vi "String_conversions.vi"() -> ()   [LabVIEW 2019]
panel:
  in  "string 2":string
  out "all lower case string":string
  in  "string":string
  out "all upper case string":string
  in  "width (-)":i16
  in  "number":i32
  out "decimal integer string":string
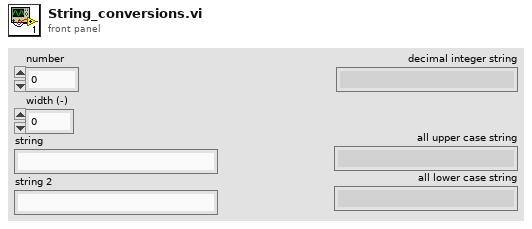
[diagram p1: front panel]
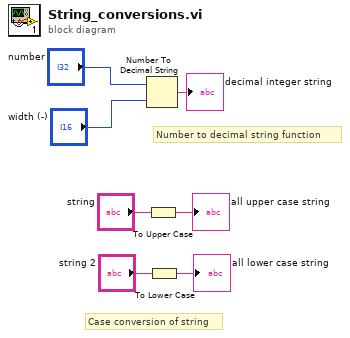
[diagram p0: block diagram]
diagram:
  # "Case conversion of string"
  # "Number to decimal string function"
  n1 = Number To Decimal String(number="number", width (-)="width (-)") -> (decimal integer string=→"decimal integer string":string)
  n2 = To Upper Case(1:"string") -> (0:→"all upper case string":string)
  n3 = To Lower Case(string="string 2") -> (all lower case string=→"all lower case string":string)
